vi "Cycle_Diag_Table_Read.vi"(7 "ERD Data In":T3[](array[typedef]) {"ERD Number" format="%.0x"}, 11 "error in (no error)":errorcluster) -> (2 "Cycle Buffer Status":T2, 3 "Diag Cycle String Out":string[][](array[string]), 8 "Cycle  Diag Array Out":T1[](array[typedef]), 15 "error out":errorcluster)   [LabVIEW 2021]
uses:
  Common/LabVIEW GEA2 Toolkit/GEA3/type defs/ERD Read Data Out.ctl
  type defs/Cycle_Diag_Buffer_Status.ctl
  type defs/Cycle_Diag.ctl
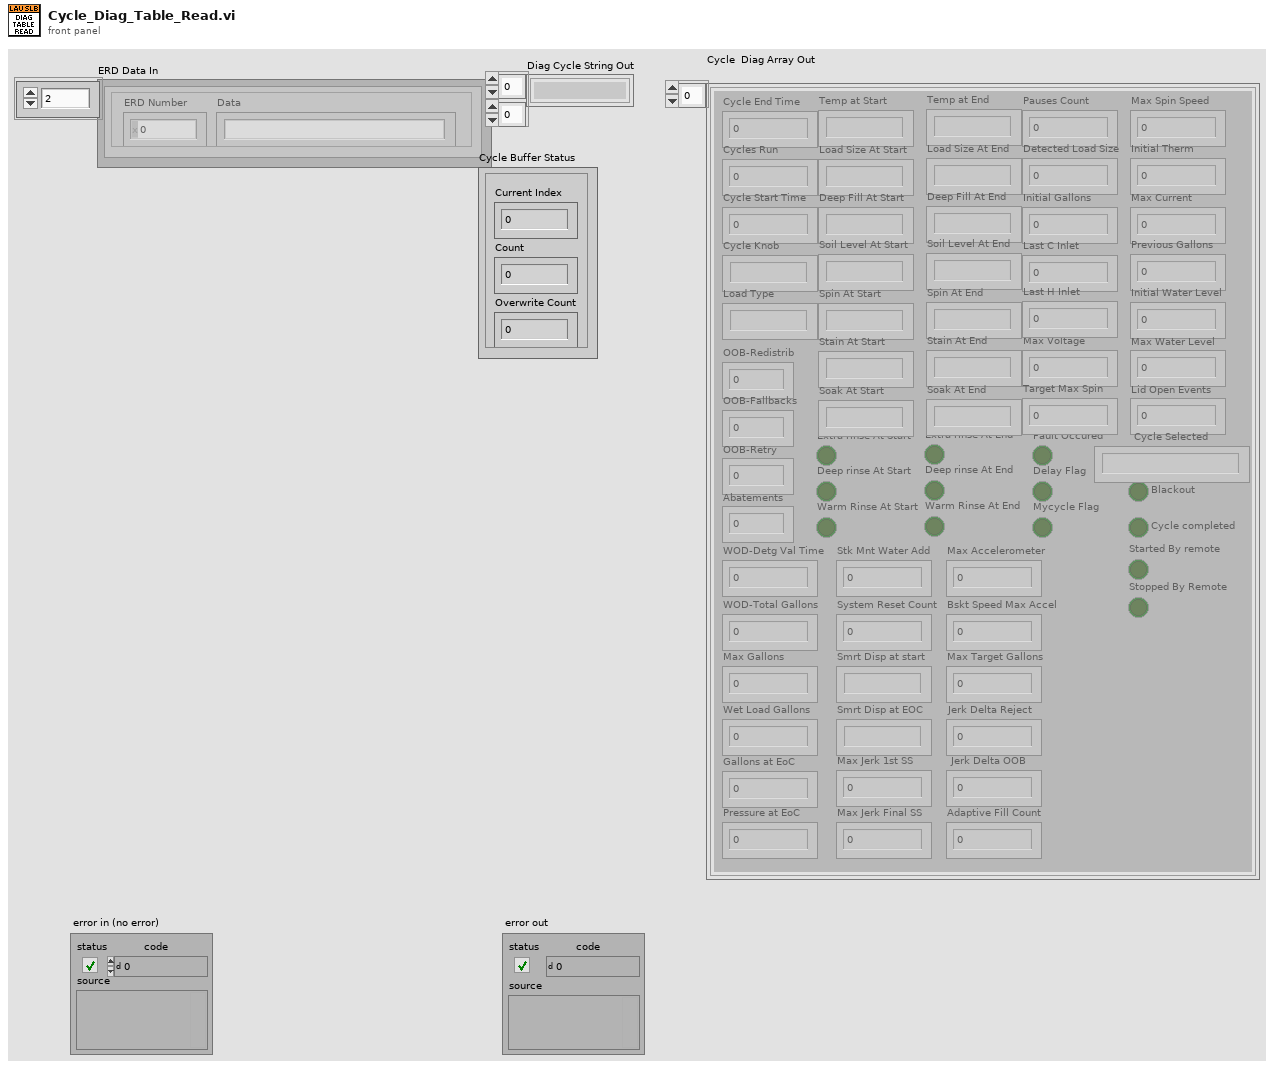
[diagram p1: front panel]
types:
  T1 = typedef "Cycle_Diag.ctl" = cluster{"Cycle End Time":u32, "Cycles Run":u32, "Cycle Start Time":u32, "Cycle Knob":string, "Load Type":string, "OOB-Redistrib":u8, "OOB-Fallbacks":u8, "OOB-Retry":u8, "Temp at Start":string, "Load Size At Start":string, "Deep Fill At Start":string, "Soil Level At Start":string, "Spin At Start":string, "Extra rinse At Start":bool, "Deep rinse At Start":bool, "Stain At Start":string, "Soak At Start":string, "Warm Rinse At Start":bool, "Temp at End":string, "Load Size At End":string, "Deep Fill At End":string, "Soil Level At End":string, "Spin At End":string, "Extra rinse At End":bool, "Deep rinse At End":bool, "Stain At End":string, "Soak At End":string, "Warm Rinse At End":bool, "Pauses Count":u8, "Fault Occured":bool, "Delay Flag":bool, "Mycycle Flag":bool, "Blackout":bool, "Cycle completed":bool, "Detected Load Size":dbl, "Initial Gallons":dbl, "Last C Inlet ":dbl, "Max Voltage":dbl, "Target Max Spin":u16, "Max Spin Speed":u16, "Initial Therm":dbl, "Max Current":dbl, "Previous Gallons":dbl, "Initial Water Level":dbl, "Max Water Level":dbl, "Abatements ":u8, "Lid Open Events":u8, "Cycle Selected":string, "Last H Inlet ":dbl, "WOD-Detg Val Time":u8, "WOD-Total Gallons":u16, "Max Gallons":u16, "Wet Load Gallons":u16, "Gallons at EoC":u16, "Pressure at EoC":u32, "Stk Mnt Water Add":u8, "Started By remote":bool, "Stopped By Remote":bool, "System Reset Count":u8, "Smrt Disp at start":string, "Smrt Disp at EOC":string, "Max Jerk 1st SS":i32, "Max Jerk Final SS":i32, "Max Accelerometer":i16, "Bskt Speed Max Accel":u16, "Max Target Gallons":u16, "Jerk Delta Reject ":u8, "Jerk Delta OOB  ":u8, "Adaptive Fill Count":u8}
  T2 = typedef "Cycle_Diag_Buffer_Status.ctl" = cluster{"Current Index":u16, "Count":u16, "Overwrite Count":u16}
  T3 = typedef "ERD Read Data Out.ctl" = cluster{"ERD Number":u16, "Data":string}
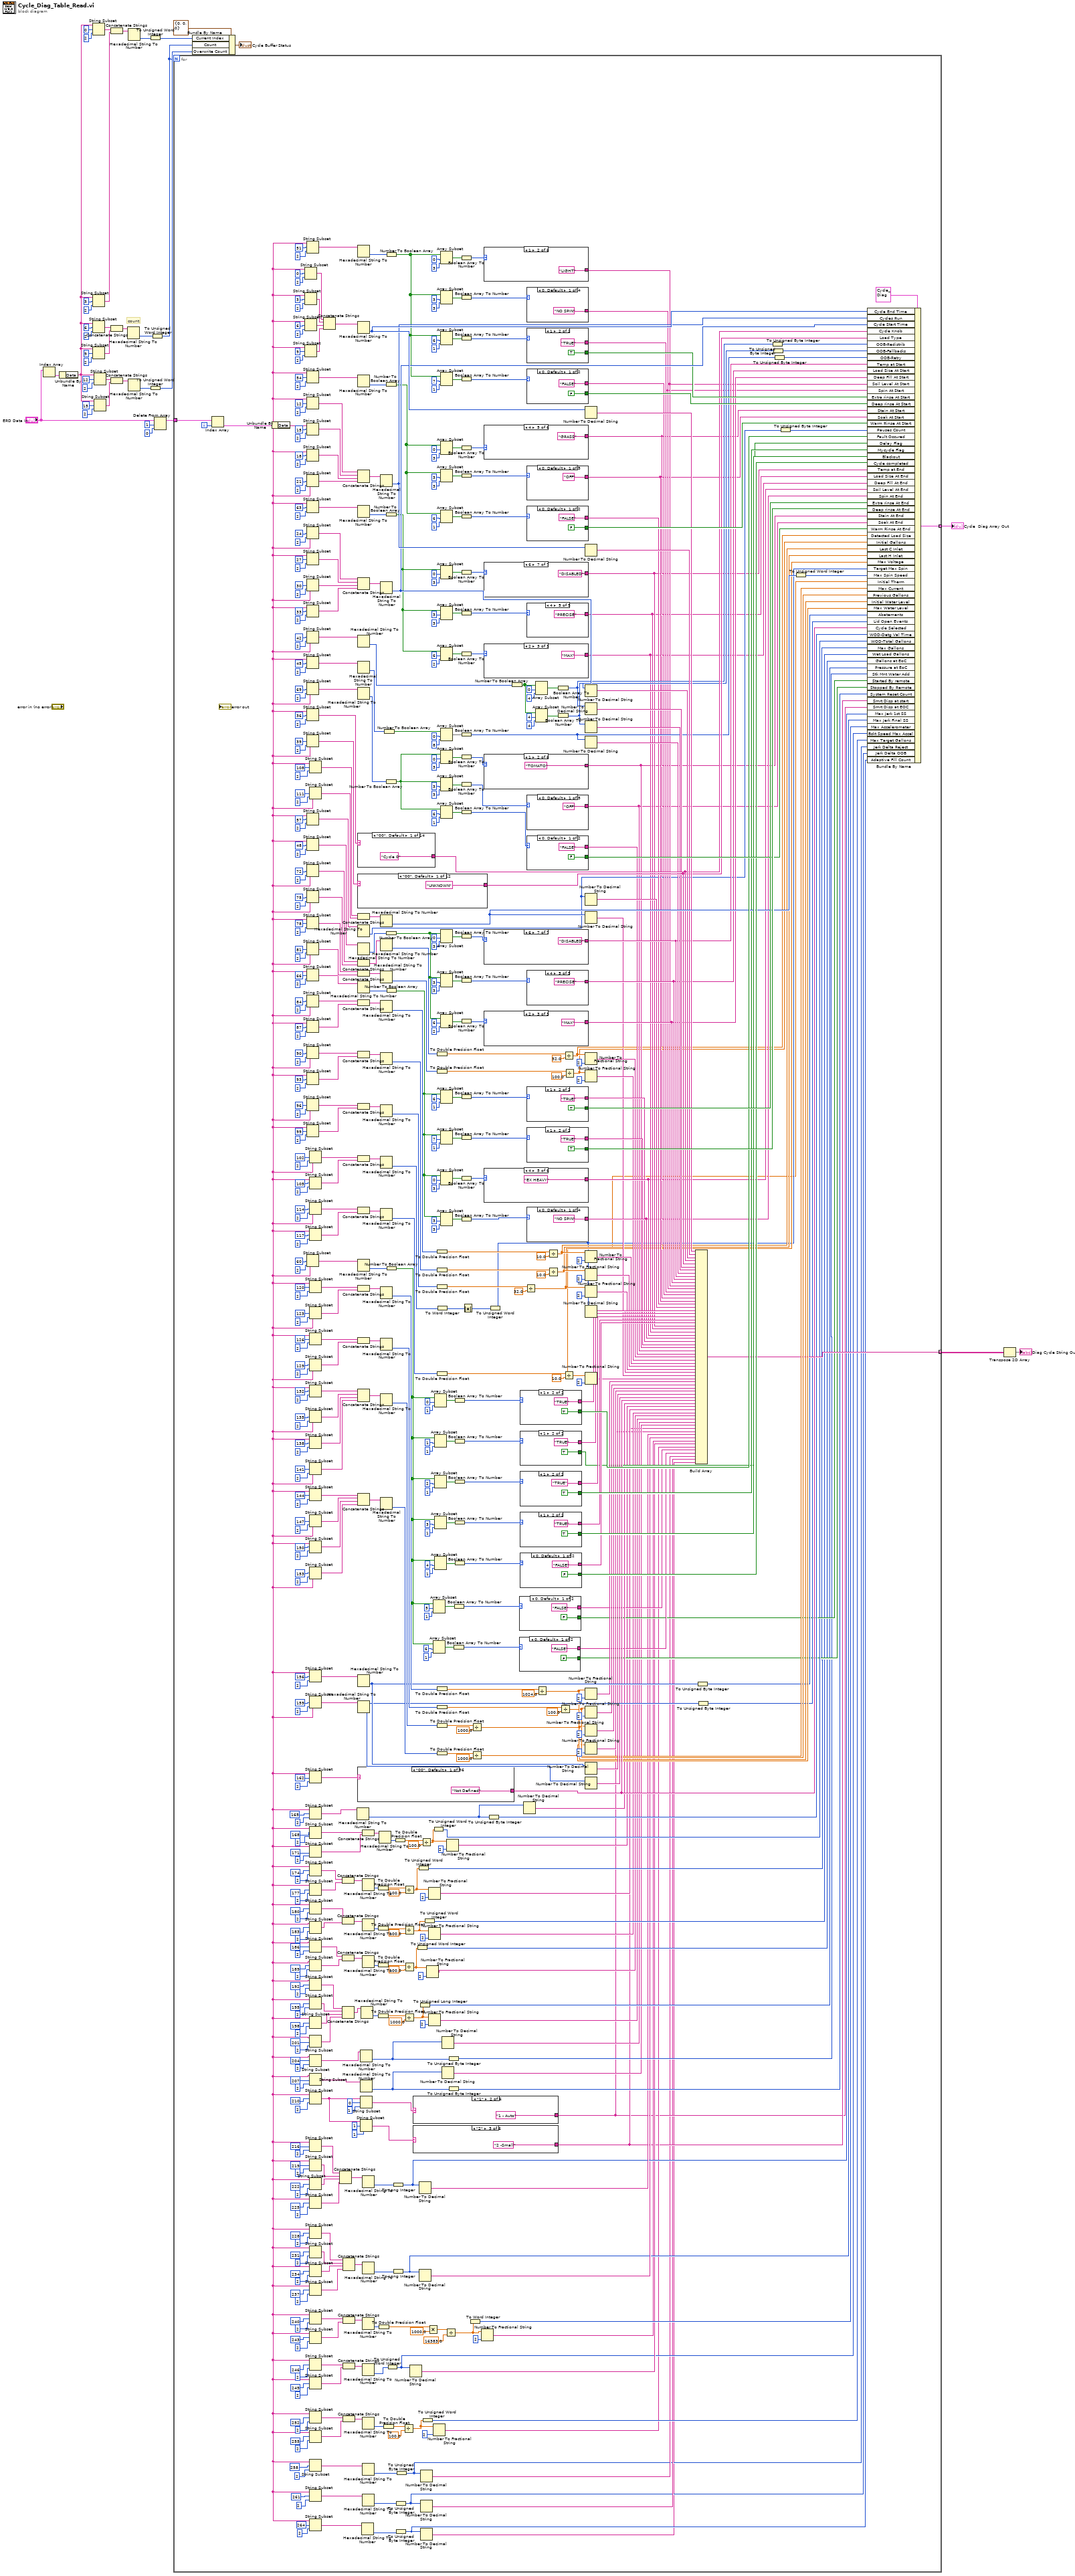
[diagram p0: block diagram]
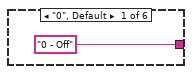
[diagram p2: hidden frame]
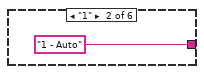
[diagram p3: hidden frame]
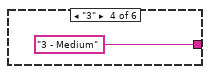
[diagram p4: hidden frame]
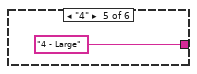
[diagram p5: hidden frame]
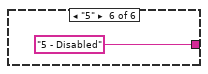
[diagram p6: hidden frame]
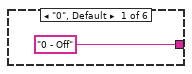
[diagram p7: hidden frame]
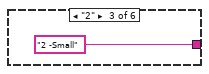
[diagram p8: hidden frame]
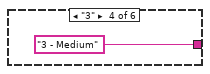
[diagram p9: hidden frame]
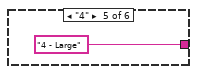
[diagram p10: hidden frame]
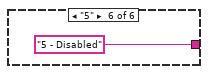
[diagram p11: hidden frame]
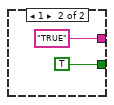
[diagram p12: hidden frame]
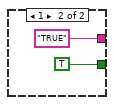
[diagram p13: hidden frame]
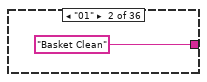
[diagram p14: hidden frame]
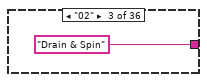
[diagram p15: hidden frame]
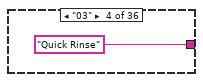
[diagram p16: hidden frame]
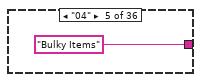
[diagram p17: hidden frame]
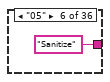
[diagram p18: hidden frame]
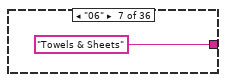
[diagram p19: hidden frame]
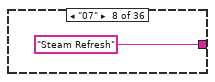
[diagram p20: hidden frame]
diagram:
  # "count"
  n1 = Index Array(array="ERD Data In") -> (element=w31:T3)  [unwired: 1 in]
  n2 = Unbundle By Name(w31) -> ("Data"=w11:string)
  n3 = String Subset(string=w11, offset (0)=0, length (rest)=2 ("length (rest)")) -> (substring=w20:string)
  n4 = String Subset(string=w11, offset (0)=3, length (rest)=2 ("length (rest)")) -> (substring=w21:string)
  n5 = String Subset(string=w11, offset (0)=6, length (rest)=2 ("length (rest)")) -> (substring=w35:string)
  n6 = String Subset(string=w11, offset (0)=9, length (rest)=2 ("length (rest)")) -> (substring=w34:string)
  n7 = String Subset(string=w11, offset (0)=12, length (rest)=2 ("length (rest)")) -> (substring=w22:string)
  n8 = String Subset(string=w11, offset (0)=15, length (rest)=2 ("length (rest)")) -> (substring=w23:string)
  n9 = Concatenate Strings(w20, w21) -> (w24:string)
  n10 = Concatenate Strings(w35, w34) -> (w33:string)
  n11 = Concatenate Strings(w22, w23) -> (w25:string)
  n12 = Hexadecimal String To Number(string=w33) -> (number=w32:u32)  [unwired: 2 in, 1 out]
  n13 = Hexadecimal String To Number(string=w24) -> (number=w26:u32)  [unwired: 2 in, 1 out]
  n14 = Hexadecimal String To Number(string=w25) -> (number=w27:u32)  [unwired: 2 in, 1 out]
  n15 = To Unsigned Word Integer(number=w26) -> (unsigned 16bit integer=w28:u16)
  n16 = To Unsigned Word Integer(number=w27) -> (unsigned 16bit integer=w29:u16)
  n17 = To Unsigned Word Integer(number=w32) -> (unsigned 16bit integer=w10:u16)
  n18 = Delete From Array(array="ERD Data In", length=1, index=0) -> (array with subset deleted=w7:T3[])  [unwired: 1 out]
  n19 = for {
    N: w10 -> [_]
    tunnel: w7 -> [w444]
    tunnel: [w441] -> w3 mode=indexing
    tunnel: [w379] -> w2 mode=indexing
    i -> [w443]
    n20 = Index Array(array=w444, index=w443) -> (element=w442:T3)
    n21 = Unbundle By Name(w442) -> ("Data"=w45:string)
    n22 = String Subset(string=w45, offset (0)=0, length (rest)=2 ("length (rest)")) -> (substring=w658:string)
    n23 = String Subset(string=w45, offset (0)=3, length (rest)=2 ("length (rest)")) -> (substring=w657:string)
    n24 = String Subset(string=w45, offset (0)=6, length (rest)=2 ("length (rest)")) -> (substring=w656:string)
    n25 = String Subset(string=w45, offset (0)=9, length (rest)=2 ("length (rest)")) -> (substring=w655:string)
    n26 = String Subset(string=w45, offset (0)=51, length (rest)=2 ("length (rest)")) -> (substring=w357:string)
    n27 = String Subset(string=w45, offset (0)=54, length (rest)=2 ("length (rest)")) -> (substring=w341:string)
    n28 = String Subset(string=w45, offset (0)=12, length (rest)=2 ("length (rest)")) -> (substring=w652:string)
    n29 = String Subset(string=w45, offset (0)=15, length (rest)=2 ("length (rest)")) -> (substring=w651:string)
    n30 = String Subset(string=w45, offset (0)=18, length (rest)=2 ("length (rest)")) -> (substring=w650:string)
    n31 = String Subset(string=w45, offset (0)=21, length (rest)=2 ("length (rest)")) -> (substring=w649:string)
    n32 = String Subset(string=w45, offset (0)=63, length (rest)=2 ("length (rest)")) -> (substring=w328:string)
    n33 = String Subset(string=w45, offset (0)=24, length (rest)=2 ("length (rest)")) -> (substring=w646:string)
    n34 = String Subset(string=w45, offset (0)=27, length (rest)=2 ("length (rest)")) -> (substring=w645:string)
    n35 = String Subset(string=w45, offset (0)=30, length (rest)=2 ("length (rest)")) -> (substring=w644:string)
    n36 = String Subset(string=w45, offset (0)=33, length (rest)=2 ("length (rest)")) -> (substring=w643:string)
    n37 = String Subset(string=w45, offset (0)=42, length (rest)=2 ("length (rest)")) -> (substring=w297:string)
    n38 = String Subset(string=w45, offset (0)=45, length (rest)=2 ("length (rest)")) -> (substring=w288:string)
    n39 = String Subset(string=w45, offset (0)=69, length (rest)=2 ("length (rest)")) -> (substring=w301:string)
    n40 = String Subset(string=w45, offset (0)=36, length (rest)=2 ("length (rest)")) -> (substring=w640:string)
    n41 = String Subset(string=w45, offset (0)=39, length (rest)=2 ("length (rest)")) -> (substring=w639:string)
    n42 = String Subset(string=w45, offset (0)=57, length (rest)=2 ("length (rest)")) -> (substring=w597:string)
    n43 = String Subset(string=w45, offset (0)=48, length (rest)=2 ("length (rest)")) -> (substring=w376:string)
    n44 = String Subset(string=w45, offset (0)=72, length (rest)=2 ("length (rest)")) -> (substring=w581:string)
    n45 = String Subset(string=w45, offset (0)=75 ("offset"), length (rest)=u32 2 ("default (0 U32)")) -> (substring=w578:string)
    n46 = String Subset(string=w45, offset (0)=78, length (rest)=2 ("length (rest)")) -> (substring=w573:string)
    n47 = String Subset(string=w45, offset (0)=81, length (rest)=2 ("length (rest)")) -> (substring=w572:string)
    n48 = String Subset(string=w45, offset (0)=66, length (rest)=2 ("length (rest)")) -> (substring=w314:string)
    n49 = String Subset(string=w45, offset (0)=84, length (rest)=2 ("length (rest)")) -> (substring=w562:string)
    n50 = String Subset(string=w45, offset (0)=87, length (rest)=2 ("length (rest)")) -> (substring=w561:string)
    n51 = String Subset(string=w45, offset (0)=90, length (rest)=2 ("length (rest)")) -> (substring=w556:string)
    n52 = String Subset(string=w45, offset (0)=93, length (rest)=2 ("length (rest)")) -> (substring=w555:string)
    n53 = String Subset(string=w45, offset (0)=96, length (rest)=2 ("length (rest)")) -> (substring=w546:string)
    n54 = String Subset(string=w45, offset (0)=99, length (rest)=2 ("length (rest)")) -> (substring=w545:string)
    n55 = String Subset(string=w45, offset (0)=60, length (rest)=2 ("length (rest)")) -> (substring=w596:string)
    n56 = String Subset(string=w45, offset (0)=108, length (rest)=2 ("length (rest)")) -> (substring=w533:string)
    n57 = String Subset(string=w45, offset (0)=111, length (rest)=2 ("length (rest)")) -> (substring=w532:string)
    n58 = String Subset(string=w45, offset (0)=102, length (rest)=2 ("length (rest)")) -> (substring=w536:string)
    n59 = String Subset(string=w45, offset (0)=105, length (rest)=2 ("length (rest)")) -> (substring=w535:string)
    n60 = String Subset(string=w45, offset (0)=114, length (rest)=2 ("length (rest)")) -> (substring=w521:string)
    n61 = String Subset(string=w45, offset (0)=117, length (rest)=2 ("length (rest)")) -> (substring=w520:string)
    n62 = String Subset(string=w45, offset (0)=120, length (rest)=2 ("length (rest)")) -> (substring=w511:string)
    n63 = String Subset(string=w45, offset (0)=123, length (rest)=2 ("length (rest)")) -> (substring=w510:string)
    n64 = String Subset(string=w45, offset (0)=126, length (rest)=2 ("length (rest)")) -> (substring=w501:string)
    n65 = String Subset(string=w45, offset (0)=129, length (rest)=2 ("length (rest)")) -> (substring=w500:string)
    n66 = String Subset(string=w45, offset (0)=132, length (rest)=2 ("length (rest)")) -> (substring=w491:string)
    n67 = String Subset(string=w45, offset (0)=135, length (rest)=2 ("length (rest)")) -> (substring=w490:string)
    n68 = String Subset(string=w45, offset (0)=138, length (rest)=2 ("length (rest)")) -> (substring=w460:string)
    n69 = String Subset(string=w45, offset (0)=141, length (rest)=2 ("length (rest)")) -> (substring=w459:string)
    n70 = String Subset(string=w45, offset (0)=144, length (rest)=2 ("length (rest)")) -> (substring=w485:string)
    n71 = String Subset(string=w45, offset (0)=147, length (rest)=2 ("length (rest)")) -> (substring=w484:string)
    n72 = String Subset(string=w45, offset (0)=150, length (rest)=2 ("length (rest)")) -> (substring=w454:string)
    n73 = String Subset(string=w45, offset (0)=153, length (rest)=2 ("length (rest)")) -> (substring=w453:string)
    n74 = String Subset(string=w45, offset (0)=156, length (rest)=2 ("length (rest)")) -> (substring=w465:string)
    n75 = String Subset(string=w45, offset (0)=159, length (rest)=2 ("length (rest)")) -> (substring=w464:string)
    n76 = String Subset(string=w45, offset (0)=162, length (rest)=2 ("length (rest)")) -> (substring=w461:string)
    n77 = String Subset(string=w45, offset (0)=165 ("length (rest)"), length (rest)=2 ("length (rest)")) -> (substring=w188:string)
    n78 = String Subset(string=w45, offset (0)=168 ("length (rest)"), length (rest)=2 ("length (rest)")) -> (substring=w172:string)
    n79 = String Subset(string=w45, offset (0)=171 ("length (rest)"), length (rest)=2 ("length (rest)")) -> (substring=w171:string)
    n80 = String Subset(string=w45, offset (0)=174 ("length (rest)"), length (rest)=2 ("length (rest)")) -> (substring=w160:string)
    n81 = String Subset(string=w45, offset (0)=177 ("length (rest)"), length (rest)=2 ("length (rest)")) -> (substring=w159:string)
    n82 = String Subset(string=w45, offset (0)=180 ("length (rest)"), length (rest)=2 ("length (rest)")) -> (substring=w149:string)
    n83 = String Subset(string=w45, offset (0)=183 ("length (rest)"), length (rest)=2 ("length (rest)")) -> (substring=w148:string)
    n84 = String Subset(string=w45, offset (0)=186 ("length (rest)"), length (rest)=2 ("length (rest)")) -> (substring=w147:string)
    n85 = String Subset(string=w45, offset (0)=189 ("length (rest)"), length (rest)=2 ("length (rest)")) -> (substring=w146:string)
    n86 = String Subset(string=w45, offset (0)=192 ("length (rest)"), length (rest)=2 ("length (rest)")) -> (substring=w144:string)
    n87 = String Subset(string=w45, offset (0)=195 ("length (rest)"), length (rest)=2 ("length (rest)")) -> (substring=w143:string)
    n88 = String Subset(string=w45, offset (0)=198 ("length (rest)"), length (rest)=2 ("length (rest)")) -> (substring=w142:string)
    n89 = String Subset(string=w45, offset (0)=201 ("length (rest)"), length (rest)=2 ("length (rest)")) -> (substring=w141:string)
    n90 = String Subset(string=w45, offset (0)=204 ("length (rest)"), length (rest)=2 ("length (rest)")) -> (substring=w134:string)
    n91 = String Subset(string=w45, offset (0)=207 ("length (rest)"), length (rest)=2 ("length (rest)")) -> (substring=w129:string)
    n92 = String Subset(string=w45, offset (0)=210 ("length (rest)"), length (rest)=2 ("length (rest)")) -> (substring=w126:string)
    n93 = String Subset(string=w45, offset (0)=216 ("length (rest)"), length (rest)=2 ("length (rest)")) -> (substring=w119:string)
    n94 = String Subset(string=w45, offset (0)=219 ("length (rest)"), length (rest)=2 ("length (rest)")) -> (substring=w118:string)
    n95 = String Subset(string=w45, offset (0)=222 ("length (rest)"), length (rest)=2 ("length (rest)")) -> (substring=w117:string)
    n96 = String Subset(string=w45, offset (0)=225 ("length (rest)"), length (rest)=2 ("length (rest)")) -> (substring=w116:string)
    n97 = String Subset(string=w45, offset (0)=228 ("length (rest)"), length (rest)=2 ("length (rest)")) -> (substring=w110:string)
    n98 = String Subset(string=w45, offset (0)=231 ("length (rest)"), length (rest)=2 ("length (rest)")) -> (substring=w109:string)
    n99 = String Subset(string=w45, offset (0)=234 ("length (rest)"), length (rest)=2 ("length (rest)")) -> (substring=w108:string)
    n100 = String Subset(string=w45, offset (0)=237 ("length (rest)"), length (rest)=2 ("length (rest)")) -> (substring=w107:string)
    n101 = String Subset(string=w45, offset (0)=240 ("length (rest)"), length (rest)=2 ("length (rest)")) -> (substring=w102:string)
    n102 = String Subset(string=w45, offset (0)=243 ("length (rest)"), length (rest)=2 ("length (rest)")) -> (substring=w101:string)
    n103 = String Subset(string=w45, offset (0)=246 ("length (rest)"), length (rest)=2 ("length (rest)")) -> (substring=w100:string)
    n104 = String Subset(string=w45, offset (0)=249 ("length (rest)"), length (rest)=2 ("length (rest)")) -> (substring=w99:string)
    n105 = String Subset(string=w45, offset (0)=252 ("length (rest)"), length (rest)=2 ("length (rest)")) -> (substring=w98:string)
    n106 = String Subset(string=w45, offset (0)=255 ("length (rest)"), length (rest)=2 ("length (rest)")) -> (substring=w97:string)
    n107 = String Subset(string=w45, offset (0)=258, length (rest)=2 ("length (rest)")) -> (substring=w50:string)
    n108 = String Subset(string=w45, offset (0)=261, length (rest)=2 ("length (rest)")) -> (substring=w53:string)
    n109 = String Subset(string=w45, offset (0)=264, length (rest)=2 ("length (rest)")) -> (substring=w42:string)
    n110 = Concatenate Strings(w658, w657, w656, w655) -> (w654:string)
    n111 = Concatenate Strings(w119, w118, w117, w116) -> (w114:string)
    n112 = Concatenate Strings(w160, w159) -> (w164:string)
    n113 = Concatenate Strings(w149, w148) -> (w157:string)
    n114 = Concatenate Strings(w147, w146) -> (w153:string)
    n115 = Concatenate Strings(w144, w143, w142, w141) -> (w137:string)
    n116 = Concatenate Strings(w110, w109, w108, w107) -> (w106:string)
    n117 = Concatenate Strings(w102, w101) -> (w95:string)
    n118 = Concatenate Strings(w100, w99) -> (w89:string)
    n119 = Concatenate Strings(w98, w97) -> (w85:string)
    n120 = Hexadecimal String To Number(string=w188) -> (number=w186:u32)  [unwired: 2 in, 1 out]
    n121 = Hexadecimal String To Number(string=w357) -> (number=w364:u32)  [unwired: 2 in, 1 out]
    n122 = Hexadecimal String To Number(string=w654) -> (number=w653:u32)  [unwired: 2 in, 1 out]
    n123 = Hexadecimal String To Number(string=w341) -> (number=w349:u32)  [unwired: 2 in, 1 out]
    n124 = Concatenate Strings(w652, w651, w650, w649) -> (w648:string)
    n125 = Hexadecimal String To Number(string=w328) -> (number=w336:u32)  [unwired: 2 in, 1 out]
    n126 = Concatenate Strings(w646, w645, w644, w643) -> (w642:string)
    n127 = Hexadecimal String To Number(string=w297) -> (number=w296:u32)  [unwired: 2 in, 1 out]
    n128 = Hexadecimal String To Number(string=w288) -> (number=w287:u32)  [unwired: 2 in, 1 out]
    n129 = Hexadecimal String To Number(string=w301) -> (number=w309:u32)  [unwired: 2 in, 1 out]
    n130 = case shown="\"00\", Default" w640 {
      tunnel: ["Cycle 0" "Cycle 1" "Cycle 2" "Cycle 3" "Cycle 4" "Cycle 5" "Cycle 6" "Cycle 7" "Cycle 8" "Cycle 9" "Cycle 10" "Cycle 11" "Cycle 12" "Cycle 13"] -> w437
      frame "00", Default {
      }
      frame "01" {
      }
      frame "02" {
      }
      frame "03" {
      }
      frame "04" {
      }
      frame "05" {
      }
      frame "06" {
      }
      frame "07" {
      }
      frame "08" {
      }
      frame "09" {
      }
      frame "0A" {
      }
      frame "0B" {
      }
      frame "0C" {
      }
      frame "0D" {
      }
    }
    n131 = case shown="\"00\", Default" w639 {
      tunnel: ["UNKNOWN" "COTTON" "SYNTHETIC" "MIXED" "WET" "LOW FLOW" "SMALL" "MEDIUM" "LARGE" "SUPER" "SUPER PLUS" "MAX"] -> w436
      frame "00", Default {
      }
      frame "01" {
      }
      frame "02" {
      }
      frame "03" {
      }
      frame "04" {
      }
      frame "05" {
      }
      frame "06" {
      }
      frame "07" {
      }
      frame "08" {
      }
      frame "09" {
      }
      frame "0A" {
      }
      frame "0B" {
      }
    }
    n132 = Concatenate Strings(w533, w532) -> (w531:string)
    n133 = Hexadecimal String To Number(string=w597) -> (number=w420:u32)  [unwired: 2 in, 1 out]
    n134 = Hexadecimal String To Number(string=w376) -> (number=w375:u32)  [unwired: 2 in, 1 out]
    n135 = Concatenate Strings(w581, w578) -> (w577:string)
    n136 = Concatenate Strings(w573, w572) -> (w571:string)
    n137 = Hexadecimal String To Number(string=w314) -> (number=w324:u32)  [unwired: 2 in, 1 out]
    n138 = Concatenate Strings(w562, w561) -> (w560:string)
    n139 = Concatenate Strings(w556, w555) -> (w554:string)
    n140 = Concatenate Strings(w546, w545) -> (w544:string)
    n141 = Concatenate Strings(w536, w535) -> (w534:string)
    n142 = Concatenate Strings(w521, w520) -> (w519:string)
    n143 = Hexadecimal String To Number(string=w596) -> (number=w595:u32)  [unwired: 2 in, 1 out]
    n144 = Concatenate Strings(w511, w510) -> (w509:string)
    n145 = Concatenate Strings(w501, w500) -> (w499:string)
    n146 = Concatenate Strings(w491, w490, w460, w459) -> (w489:string)
    n147 = Concatenate Strings(w485, w484, w454, w453) -> (w483:string)
    n148 = Hexadecimal String To Number(string=w465) -> (number=w463:u32)  [unwired: 2 in, 1 out]
    n149 = Hexadecimal String To Number(string=w464) -> (number=w462:u32)  [unwired: 2 in, 1 out]
    n150 = case shown="\"00\", Default" w461 {
      tunnel: ["Not Defined" "Basket Clean" "Drain & Spin" "Quick Rinse" "Bulky Items" "Sanitize" "Towels & Sheets" "Steam Refresh" "Normal/Mixed" "Whites" "Dark Colors" "Jeans" "Hand Wash" "Delicates" "Speed Wash" "Heavy Duty" "Allergen" "Power Clean" "Rinse & Spin" "Single Item" "Colors" "Cold Wash" "Cottons" "Easy Care" "Active Wear" "Timed Dry" "Dewrinkle" "Air Fluff" "Steam Refresh" "Steam Dewrinkle" "Speed Dry" "Mixed" "Quick Dry" "Casuals" "Warm Up" "Energy Saver"] -> w387
      frame "00", Default {
      }
      frame "01" {
      }
      frame "02" {
      }
      frame "03" {
      }
      frame "04" {
      }
      frame "05" {
      }
      frame "06" {
      }
      frame "07" {
      }
      frame "08" {
      }
      frame "09" {
      }
      frame "0A" {
      }
      frame "0B" {
      }
      frame "0C" {
      }
      frame "0D" {
      }
      frame "0E" {
      }
      frame "0F" {
      }
      frame "10" {
      }
      frame "11" {
      }
      frame "12" {
      }
      frame "13" {
      }
      frame "14" {
      }
      frame "15" {
      }
      frame "80" {
      }
      frame "81" {
      }
      frame "82" {
      }
      frame "83" {
      }
      frame "84" {
      }
      frame "85" {
      }
      frame "86" {
      }
      frame "87" {
      }
      frame "88" {
      }
      frame "89" {
      }
      frame "8A" {
      }
      frame "8B" {
      }
      frame "8C" {
      }
      frame "8D" {
      }
    }
    n151 = Hexadecimal String To Number(string=w134) -> (number=w133:u32)  [unwired: 2 in, 1 out]
    n152 = Hexadecimal String To Number(string=w129) -> (number=w130:u32)  [unwired: 2 in, 1 out]
    n153 = String Subset(string=w126, offset (0)=0, length (rest)=1 ("length (rest)")) -> (substring=w121:string)
    n154 = String Subset(string=w126, offset (0)=1, length (rest)=1 ("length (rest)")) -> (substring=w120:string)
    n155 = Hexadecimal String To Number(string=w137) -> (number=w140:u32)  [unwired: 2 in, 1 out]
    n156 = Hexadecimal String To Number(string=w42) -> (number=w41:u32)  [unwired: 2 in, 1 out]
    n157 = Concatenate Strings(w172, w171) -> (w170:string)
    n158 = Hexadecimal String To Number(string=w164) -> (number=w163:u32)  [unwired: 2 in, 1 out]
    n159 = Hexadecimal String To Number(string=w157) -> (number=w156:u32)  [unwired: 2 in, 1 out]
    n160 = Hexadecimal String To Number(string=w153) -> (number=w152:u32)  [unwired: 2 in, 1 out]
    n161 = Hexadecimal String To Number(string=w95) -> (number=w96:u32)  [unwired: 2 in, 1 out]
    n162 = Hexadecimal String To Number(string=w89) -> (number=w60:u32)  [unwired: 2 in, 1 out]
    n163 = Hexadecimal String To Number(string=w85) -> (number=w86:u32)  [unwired: 2 in, 1 out]
    n164 = Hexadecimal String To Number(string=w50) -> (number=w52:u32)  [unwired: 2 in, 1 out]
    n165 = Hexadecimal String To Number(string=w53) -> (number=w51:u32)  [unwired: 2 in, 1 out]
    n166 = Hexadecimal String To Number(string=w114) -> (number=w113:u32)  [unwired: 2 in, 1 out]
    n167 = Hexadecimal String To Number(string=w106) -> (number=w105:u32)  [unwired: 2 in, 1 out]
    n168 = To Double Precision Float(number=w163) -> (double precision float=w162:dbl)
    n169 = To Double Precision Float(number=w156) -> (double precision float=w155:dbl)
    n170 = To Double Precision Float(number=w152) -> (double precision float=w151:dbl)
    n171 = To Double Precision Float(number=w140) -> (double precision float=w139:dbl)
    n172 = To Double Precision Float(number=w96) -> (double precision float=w94:dbl)
    n173 = Hexadecimal String To Number(string=w170) -> (number=w169:u32)  [unwired: 2 in, 1 out]
    n174 = Hexadecimal String To Number(string=w648) -> (number=w647:u32)  [unwired: 2 in, 1 out]
    n175 = Hexadecimal String To Number(string=w642) -> (number=w641:u32)  [unwired: 2 in, 1 out]
    n176 = Hexadecimal String To Number(string=w531) -> (number=w530:u32)  [unwired: 2 in, 1 out]
    n177 = Hexadecimal String To Number(string=w577) -> (number=w584:u32)  [unwired: 2 in, 1 out]
    n178 = Hexadecimal String To Number(string=w571) -> (number=w570:u32)  [unwired: 2 in, 1 out]
    n179 = Hexadecimal String To Number(string=w560) -> (number=w559:u32)  [unwired: 2 in, 1 out]
    n180 = Hexadecimal String To Number(string=w554) -> (number=w553:u32)  [unwired: 2 in, 1 out]
    n181 = Hexadecimal String To Number(string=w544) -> (number=w543:u32)  [unwired: 2 in, 1 out]
    n182 = Hexadecimal String To Number(string=w534) -> (number=w446:u32)  [unwired: 2 in, 1 out]
    n183 = Hexadecimal String To Number(string=w519) -> (number=w518:u32)  [unwired: 2 in, 1 out]
    n184 = Hexadecimal String To Number(string=w509) -> (number=w508:u32)  [unwired: 2 in, 1 out]
    n185 = Hexadecimal String To Number(string=w499) -> (number=w498:u32)  [unwired: 2 in, 1 out]
    n186 = Hexadecimal String To Number(string=w489) -> (number=w488:u32)  [unwired: 2 in, 1 out]
    n187 = Hexadecimal String To Number(string=w483) -> (number=w482:u32)  [unwired: 2 in, 1 out]
    n188 = To Double Precision Float(number=w86) -> (double precision float=w84:dbl)
    n189 = Number To Boolean Array(number=w287) -> (Boolean array=w286:bool[])
    n190 = Number To Boolean Array(number=w349) -> (Boolean array=w348:bool[])
    n191 = Number To Boolean Array(number=w336) -> (Boolean array=w335:bool[])
    n192 = Number To Boolean Array(number=w309) -> (Boolean array=w308:bool[])
    n193 = Number To Boolean Array(number=w375) -> (Boolean array=w374:bool[])
    n194 = Number To Boolean Array(number=w364) -> (Boolean array=w356:bool[])
    n195 = Number To Boolean Array(number=w324) -> (Boolean array=w317:bool[])
    n196 = Number To Boolean Array(number=w595) -> (Boolean array=w176:bool[])
    n197 = To Unsigned Word Integer(number=w60) -> (unsigned 16bit integer=w87:u16)
    n198 = To Long Integer(number=w113) -> (32bit integer=w111:i32)
    n199 = To Long Integer(number=w105) -> (32bit integer=w103:i32)
    n200 = To Double Precision Float(number=w169) -> (double precision float=w168:dbl)
    n201 = To Unsigned Byte Integer(number=w51) -> (unsigned 8bit integer=w46:u8)
    n202 = To Unsigned Byte Integer(number=w41) -> (unsigned 8bit integer=w40:u8)
    n203 = To Unsigned Byte Integer(number=w52) -> (unsigned 8bit integer=w47:u8)
    n204 = Divide(x=w84, y=100.0) -> (x/y=w68:dbl)
    n205 = Divide(x=w162, y=100.0) -> (x/y=w79:dbl)
    n206 = Divide(x=w155, y=100.0) -> (x/y=w76:dbl)
    n207 = Divide(x=w151, y=100.0) -> (x/y=w75:dbl)
    n208 = Divide(x=w139, y=1000.0) -> (x/y=w72:dbl)
    n209 = Number To Decimal String(number=w87) -> (decimal integer string=w88:string)  [unwired: 1 in]
    n210 = case shown="\"2\"" w120 {
      tunnel: ["0 - Off" "1 - Auto" "2 -Small" "3 - Medium" "4 - Large" "5 - Disabled"] -> w59
      frame "0", Default {
      }
      frame "1" {
      }
      frame "2" {
      }
      frame "3" {
      }
      frame "4" {
      }
      frame "5" {
      }
    }
    n211 = case shown="\"1\"" w121 {
      tunnel: ["0 - Off" "1 - Auto" "2 -Small" "3 - Medium" "4 - Large" "5 - Disabled"] -> w58
      frame "0", Default {
      }
      frame "1" {
      }
      frame "2" {
      }
      frame "3" {
      }
      frame "4" {
      }
      frame "5" {
      }
    }
    n212 = To Unsigned Word Integer(number=w75) -> (unsigned 16bit integer=w135:u16)
    n213 = To Unsigned Word Integer(number=w79) -> (unsigned 16bit integer=w158:u16)
    n214 = To Unsigned Long Integer(number=w72) -> (unsigned 32bit integer=w136:u32)
    n215 = Number To Decimal String(number=w111) -> (decimal integer string=w112:string)  [unwired: 1 in]
    n216 = Number To Decimal String(number=w103) -> (decimal integer string=w104:string)  [unwired: 1 in]
    n217 = Number To Decimal String(number=w47) -> (decimal integer string=w49:string)  [unwired: 1 in]
    n218 = Number To Decimal String(number=w46) -> (decimal integer string=w48:string)  [unwired: 1 in]
    n219 = Number To Decimal String(number=w40) -> (decimal integer string=w39:string)  [unwired: 1 in]
    n220 = Divide(x=w168, y=100.0) -> (x/y=w81:dbl)
    n221 = To Unsigned Word Integer(number=w68) -> (unsigned 16bit integer=w82:u16)
    n222 = To Unsigned Word Integer(number=w76) -> (unsigned 16bit integer=w145:u16)
    n223 = Number To Fractional String(number=w75, precision (6)=i16 2) -> (F-format string=w74:string)  [unwired: 2 in]
    n224 = Multiply(x=w94, y=1000.0) -> (x*y=w92:dbl)
    n225 = Number To Fractional String(number=w72, precision (6)=i16 2) -> (F-format string=w73:string)  [unwired: 2 in]
    n226 = Number To Fractional String(number=w79, precision (6)=i16 2) -> (F-format string=w78:string)  [unwired: 2 in]
    n227 = Number To Fractional String(number=w76, precision (6)=i16 2) -> (F-format string=w77:string)  [unwired: 2 in]
    n228 = To Unsigned Word Integer(number=w81) -> (unsigned 16bit integer=w166:u16)
    n229 = Array Subset(array=w176, index=6, length=1) -> (w177:bool[])
    n230 = Number To Fractional String(number=w68, precision (6)=i16 2) -> (F-format string=w69:string)  [unwired: 2 in]
    n231 = Array Subset(array=w176, index=5, length=1) -> (w181:bool[])
    n232 = Array Subset(array=w176, index=0, length=1) -> (w272:bool[])
    n233 = Array Subset(array=w176, index=1, length=1) -> (w270:bool[])
    n234 = Array Subset(array=w176, index=2, length=1) -> (w269:bool[])
    n235 = Array Subset(array=w176, index=3, length=1) -> (w268:bool[])
    n236 = Array Subset(array=w176, index=4, length=1) -> (w267:bool[])
    n237 = To Double Precision Float(number=w584) -> (double precision float=w583:dbl)
    n238 = To Double Precision Float(number=w570) -> (double precision float=w569:dbl)
    n239 = To Double Precision Float(number=w559) -> (double precision float=w558:dbl)
    n240 = To Double Precision Float(number=w553) -> (double precision float=w552:dbl)
    n241 = To Double Precision Float(number=w543) -> (double precision float=w542:dbl)
    n242 = To Word Integer(number=w446) -> (16bit integer=w448:i16)
    n243 = To Double Precision Float(number=w518) -> (double precision float=w517:dbl)
    n244 = To Double Precision Float(number=w508) -> (double precision float=w507:dbl)
    n245 = To Double Precision Float(number=w498) -> (double precision float=w497:dbl)
    n246 = To Double Precision Float(number=w488) -> (double precision float=w487:dbl)
    n247 = To Double Precision Float(number=w482) -> (double precision float=w481:dbl)
    n248 = Array Subset(array=w356, index=0, length=3) -> (w353:bool[])
    n249 = Array Subset(array=w356, index=3, length=3) -> (w352:bool[])
    n250 = Array Subset(array=w356, index=6, length=1) -> (w351:bool[])
    n251 = Array Subset(array=w356, index=7, length=1) -> (w350:bool[])
    n252 = Array Subset(array=w348, index=0, length=3) -> (w339:bool[])
    n253 = Array Subset(array=w348, index=3, length=3) -> (w338:bool[])
    n254 = Array Subset(array=w348, index=6, length=1) -> (w337:bool[])
    n255 = Array Subset(array=w335, index=0, length=3) -> (w327:bool[])
    n256 = Array Subset(array=w335, index=3, length=3) -> (w326:bool[])
    n257 = Array Subset(array=w335, index=6, length=2) -> (w325:bool[])
    n258 = Array Subset(array=w286, index=0, length=8) -> (w283:bool[])
    n259 = Array Subset(array=w308, index=0, length=3) -> (w300:bool[])
    n260 = Array Subset(array=w308, index=3, length=3) -> (w299:bool[])
    n261 = Array Subset(array=w308, index=6, length=1) -> (w298:bool[])
    n262 = Array Subset(array=w374, index=0, length=3) -> (w367:bool[])
    n263 = Array Subset(array=w374, index=3, length=3) -> (w366:bool[])
    n264 = Array Subset(array=w374, index=6, length=2) -> (w365:bool[])
    n265 = Array Subset(array=w317, index=6, length=1) -> (w311:bool[])
    n266 = Array Subset(array=w317, index=7, length=1) -> (w310:bool[])
    n267 = Array Subset(array=w317, index=0, length=3) -> (w313:bool[])
    n268 = Array Subset(array=w317, index=3, length=3) -> (w312:bool[])
    n269 = Number To Decimal String(number=w133) -> (decimal integer string=w132:string)  [unwired: 1 in]
    n270 = Number To Decimal String(number=w130) -> (decimal integer string=w128:string)  [unwired: 1 in]
    n271 = Divide(x=w92, y=16383.0) -> (x/y=w70:dbl)
    n272 = Number To Fractional String(number=w81, precision (6)=i16 2) -> (F-format string=w80:string)  [unwired: 2 in]
    n273 = To Unsigned Byte Integer(number=w133) -> (unsigned 8bit integer=w131:u8)
    n274 = To Unsigned Byte Integer(number=w130) -> (unsigned 8bit integer=w127:u8)
    n275 = Boolean Array To Number(Boolean array=w177) -> (number=w180:u32)
    n276 = Boolean Array To Number(Boolean array=w181) -> (number=w184:u32)
    n277 = Boolean Array To Number(Boolean array=w272) -> (number=w594:u32)
    n278 = Boolean Array To Number(Boolean array=w270) -> (number=w593:u32)
    n279 = Boolean Array To Number(Boolean array=w269) -> (number=w592:u32)
    n280 = Boolean Array To Number(Boolean array=w268) -> (number=w591:u32)
    n281 = Boolean Array To Number(Boolean array=w267) -> (number=w590:u32)
    n282 = Boolean Array To Number(Boolean array=w353) -> (number=w630:u32)
    n283 = Boolean Array To Number(Boolean array=w352) -> (number=w629:u32)
    n284 = Boolean Array To Number(Boolean array=w351) -> (number=w628:u32)
    n285 = Boolean Array To Number(Boolean array=w350) -> (number=w627:u32)
    n286 = Boolean Array To Number(Boolean array=w339) -> (number=w624:u32)
    n287 = Boolean Array To Number(Boolean array=w338) -> (number=w623:u32)
    n288 = Boolean Array To Number(Boolean array=w337) -> (number=w622:u32)
    n289 = Boolean Array To Number(Boolean array=w327) -> (number=w614:u32)
    n290 = Boolean Array To Number(Boolean array=w326) -> (number=w613:u32)
    n291 = Boolean Array To Number(Boolean array=w325) -> (number=w612:u32)
    n292 = Boolean Array To Number(Boolean array=w283) -> (number=w430:u32)
    n293 = Boolean Array To Number(Boolean array=w300) -> (number=w607:u32)
    n294 = Boolean Array To Number(Boolean array=w299) -> (number=w606:u32)
    n295 = Boolean Array To Number(Boolean array=w298) -> (number=w605:u32)
    n296 = Boolean Array To Number(Boolean array=w367) -> (number=w445:u32)
    n297 = Boolean Array To Number(Boolean array=w366) -> (number=w632:u32)
    n298 = Boolean Array To Number(Boolean array=w365) -> (number=w631:u32)
    n299 = Boolean Array To Number(Boolean array=w311) -> (number=w609:u32)
    n300 = Boolean Array To Number(Boolean array=w310) -> (number=w608:u32)
    n301 = Boolean Array To Number(Boolean array=w313) -> (number=w611:u32)
    n302 = Boolean Array To Number(Boolean array=w312) -> (number=w610:u32)
    n303 = Absolute Value(x=w448) -> (abs(x)=w447:i16)
    n304 = To Word Integer(number=w70) -> (16bit integer=w90:i16)
    n305 = Divide(x=w487, y=1000.0) -> (x/y=w381:dbl)
    n306 = Divide(x=w481, y=1000.0) -> (x/y=w380:dbl)
    n307 = Number To Fractional String(number=w70, precision (6)=i16 2) -> (F-format string=w71:string)  [unwired: 2 in]
    n308 = case shown="1" w630 {
      tunnel: ["EXTRA LIGHT" "LIGHT" "NORMAL" "HEAVY" "EX HEAVY" "DISABLED"] -> w426
      frame 0, Default {
      }
      frame 1 {
      }
      frame 2 {
      }
      frame 3 {
      }
      frame 4 {
      }
      frame 5 {
      }
    }
    n309 = case shown="4" w624 {
      tunnel: ["OFF" "TOMATO" "WINE" "BLOOD" "GRASS" "DIRT"] -> w340
      frame 0, Default {
      }
      frame 1 {
      }
      frame 2 {
      }
      frame 3 {
      }
      frame 4 {
      }
      frame 5 {
      }
    }
    n310 = case shown="6" w614 {
      tunnel: ["TAP COLD" "COLD" "COOL" "COLORS" "WARM" "HOT" "DISABLED"] -> w412
      frame 0, Default {
      }
      frame 1 {
      }
      frame 2 {
      }
      frame 3 {
      }
      frame 4 {
      }
      frame 5 {
      }
      frame 6 {
      }
    }
    n311 = case shown="2" w612 {
      tunnel: ["OFF" "INCREMENTAL" "MAX"] -> w410
      frame 0, Default {
      }
      frame 1 {
      }
      frame 2 {
      }
    }
    n312 = case shown="1" w607 {
      tunnel: ["OFF" "TOMATO" "WINE" "BLOOD" "GRASS" "DIRT"] -> w405
      frame 0, Default {
      }
      frame 1 {
      }
      frame 2 {
      }
      frame 3 {
      }
      frame 4 {
      }
      frame 5 {
      }
    }
    n313 = case shown="6" w445 {
      tunnel: ["TAP COLD" "COLD" "COOL" "COLORS" "WARM" "HOT" "DISABLED"] -> w429
      frame 0, Default {
      }
      frame 1 {
      }
      frame 2 {
      }
      frame 3 {
      }
      frame 4 {
      }
      frame 5 {
      }
      frame 6 {
      }
    }
    n314 = case shown="2" w631 {
      tunnel: ["OFF" "INCREMENTAL" "MAX"] -> w427
      frame 0, Default {
      }
      frame 1 {
      }
      frame 2 {
      }
    }
    n315 = case shown="4" w611 {
      tunnel: ["EXTRA LIGHT" "LIGHT" "NORMAL" "HEAVY" "EX HEAVY" "DISABLED"] -> w409
      frame 0, Default {
      }
      frame 1 {
      }
      frame 2 {
      }
      frame 3 {
      }
      frame 4 {
      }
      frame 5 {
      }
    }
    n316 = To Unsigned Byte Integer(number=w186) -> (unsigned 8bit integer=w185:u8)
    n317 = To Unsigned Word Integer(number=w447) -> (unsigned 16bit integer=w256:u16)
    n318 = Number To Boolean Array(number=w296) -> (Boolean array=w291:bool[])
    n319 = case shown="0, Default" w180 {
      tunnel: [FALSE TRUE] -> w165
      tunnel: ["FALSE" "TRUE"] -> w174
      frame 0, Default {
      }
      frame 1 {
      }
    }
    n320 = case shown="0, Default" w184 {
      tunnel: [FALSE TRUE] -> w173
      tunnel: ["FALSE" "TRUE"] -> w175
      frame 0, Default {
      }
      frame 1 {
      }
    }
    n321 = case shown="1" w594 {
      tunnel: [FALSE TRUE] -> w589
      tunnel: ["FALSE" "TRUE"] -> w417
      frame 0, Default {
      }
      frame 1 {
      }
    }
    n322 = case shown="1" w593 {
      tunnel: [FALSE TRUE] -> w271
      tunnel: ["FALSE" "TRUE"] -> w416
      frame 0, Default {
      }
      frame 1 {
      }
    }
    n323 = case shown="1" w592 {
      tunnel: [FALSE TRUE] -> w418
      tunnel: ["FALSE" "TRUE"] -> w415
      frame 0, Default {
      }
      frame 1 {
      }
    }
    n324 = case shown="1" w591 {
      tunnel: [FALSE TRUE] -> w588
      tunnel: ["FALSE" "TRUE"] -> w414
      frame 0, Default {
      }
      frame 1 {
      }
    }
    n325 = case shown="0, Default" w590 {
      tunnel: [FALSE TRUE] -> w587
      tunnel: ["FALSE" "TRUE"] -> w413
      frame 0, Default {
      }
      frame 1 {
      }
    }
    n326 = Number To Decimal String(number=w186) -> (decimal integer string=w187:string)  [unwired: 1 in]
    n327 = Divide(x=w542, y=32.0) -> (x/y=w384:dbl)
    n328 = case shown="0, Default" w629 {
      tunnel: ["NO SPIN" "NORMAL" "MORE" "MAX"] -> w425
      frame 0, Default {
      }
      frame 1 {
      }
      frame 2 {
      }
      frame 3 {
      }
    }
    n329 = case shown="1" w628 {
      tunnel: [FALSE TRUE] -> w626
      tunnel: ["FALSE" "TRUE"] -> w424
      frame 0, Default {
      }
      frame 1 {
      }
    }
    n330 = case shown="0, Default" w627 {
      tunnel: [FALSE TRUE] -> w625
      tunnel: ["FALSE" "TRUE"] -> w423
      frame 0, Default {
      }
      frame 1 {
      }
    }
    n331 = case shown="0, Default" w623 {
      tunnel: ["OFF" "15 MIN" "30 MIN" "60 MIN" "2 HOURS"] -> w422
      frame 0, Default {
      }
      frame 1 {
      }
      frame 2 {
      }
      frame 3 {
      }
      frame 4 {
      }
    }
    n332 = case shown="0, Default" w622 {
      tunnel: [FALSE TRUE] -> w621
      tunnel: ["FALSE" "TRUE"] -> w421
      frame 0, Default {
      }
      frame 1 {
      }
    }
    n333 = case shown="4" w613 {
      tunnel: ["SMALL" "MEDIUM" "LARGE" "SUPER" "PRECISE"] -> w411
      frame 0, Default {
      }
      frame 1 {
      }
      frame 2 {
      }
      frame 3 {
      }
      frame 4 {
      }
    }
    n334 = case shown="0, Default" w606 {
      tunnel: ["OFF" "15 MIN" "30 MIN" "60 MIN" "2 HOURS"] -> w404
      frame 0, Default {
      }
      frame 1 {
      }
      frame 2 {
      }
      frame 3 {
      }
      frame 4 {
      }
    }
    n335 = case shown="0, Default" w605 {
      tunnel: [FALSE TRUE] -> w602
      tunnel: ["FALSE" "TRUE"] -> w403
      frame 0, Default {
      }
      frame 1 {
      }
    }
    n336 = case shown="4" w632 {
      tunnel: ["SMALL" "MEDIUM" "LARGE" "SUPER" "PRECISE"] -> w428
      frame 0, Default {
      }
      frame 1 {
      }
      frame 2 {
      }
      frame 3 {
      }
      frame 4 {
      }
    }
    n337 = case shown="1" w609 {
      tunnel: [FALSE TRUE] -> w604
      tunnel: ["FALSE" "TRUE"] -> w407
      frame 0, Default {
      }
      frame 1 {
      }
    }
    n338 = case shown="1" w608 {
      tunnel: [FALSE TRUE] -> w603
      tunnel: ["FALSE" "TRUE"] -> w406
      frame 0, Default {
      }
      frame 1 {
      }
    }
    n339 = case shown="0, Default" w610 {
      tunnel: ["NO SPIN" "NORMAL" "MORE" "MAX"] -> w408
      frame 0, Default {
      }
      frame 1 {
      }
      frame 2 {
      }
      frame 3 {
      }
    }
    n340 = Array Subset(array=w291, index=0, length=4) -> (w290:bool[])
    n341 = Array Subset(array=w291, index=4, length=4) -> (w289:bool[])
    n342 = Divide(x=w507, y=1024.0) -> (x/y=w383:dbl)
    n343 = Divide(x=w558, y=10.0) -> (x/y=w386:dbl)
    n344 = Divide(x=w552, y=10.0) -> (x/y=w385:dbl)
    n345 = Boolean Array To Number(Boolean array=w290) -> (number=w435:u32)
    n346 = Boolean Array To Number(Boolean array=w289) -> (number=w433:u32)
    n347 = Divide(x=w497, y=100.0) -> (x/y=w382:dbl)
    n348 = Divide(x=w583, y=32.0) -> (x/y=w402:dbl)
    n349 = Divide(x=w517, y=10.0) -> (x/y=w115:dbl)
    n350 = Divide(x=w569, y=100.0) -> (x/y=w378:dbl)
    n351 = Number To Decimal String(number=w653) -> (decimal integer string=w440:string)  [unwired: 1 in]
    n352 = Number To Decimal String(number=w647) -> (decimal integer string=w439:string)  [unwired: 1 in]
    n353 = Number To Decimal String(number=w641) -> (decimal integer string=w438:string)  [unwired: 1 in]
    n354 = Number To Decimal String(number=w435) -> (decimal integer string=w434:string)  [unwired: 1 in]
    n355 = Number To Decimal String(number=w433) -> (decimal integer string=w432:string)  [unwired: 1 in]
    n356 = Number To Decimal String(number=w430) -> (decimal integer string=w431:string)  [unwired: 1 in]
    n357 = Number To Decimal String(number=w420) -> (decimal integer string=w419:string)  [unwired: 1 in]
    n358 = Number To Decimal String(number=w530) -> (decimal integer string=w395:string)  [unwired: 1 in]
    n359 = Number To Fractional String(number=w402, precision (6)=i16 2) -> (F-format string=w401:string)  [unwired: 2 in]
    n360 = Number To Fractional String(number=w378, precision (6)=i16 2) -> (F-format string=w400:string)  [unwired: 2 in]
    n361 = Number To Fractional String(number=w386, precision (6)=i16 2) -> (F-format string=w399:string)  [unwired: 2 in]
    n362 = Number To Fractional String(number=w385, precision (6)=i16 2) -> (F-format string=w398:string)  [unwired: 2 in]
    n363 = Number To Fractional String(number=w384, precision (6)=i16 2) -> (F-format string=w397:string)  [unwired: 2 in]
    n364 = Number To Decimal String(number=w256) -> (decimal integer string=w396:string)  [unwired: 1 in]
    n365 = Number To Fractional String(number=w115, precision (6)=i16 2) -> (F-format string=w394:string)  [unwired: 2 in]
    n366 = Number To Fractional String(number=w383, precision (6)=i16 2) -> (F-format string=w393:string)  [unwired: 2 in]
    n367 = Number To Fractional String(number=w382, precision (6)=i16 2) -> (F-format string=w392:string)  [unwired: 2 in]
    n368 = Number To Fractional String(number=w381, precision (6)=i16 2) -> (F-format string=w391:string)  [unwired: 2 in]
    n369 = Number To Fractional String(number=w380, precision (6)=i16 2) -> (F-format string=w390:string)  [unwired: 2 in]
    n370 = Number To Decimal String(number=w463) -> (decimal integer string=w389:string)  [unwired: 1 in]
    n371 = Number To Decimal String(number=w462) -> (decimal integer string=w388:string)  [unwired: 1 in]
    n372 = Build Array(w440, w439, w438, w437, w436, w434, w432, w431, w429, w428, w427, w426, w425, w424, w423, w340, w422, w421, w419, w417, w416, w415, w414, w413, w412, w411, w410, w409, w408, w407, w406, w405, w404, w403, w401, w400, w399, w398, w397, w396, w395, w394, w393, w392, w391, w390, w389, w388, w387, w187, w80, w78, w77, w74, w73, w132, w128, w59, w58, w112, w104, w71, w88, w69, w175, w174, w49, w48, w39) -> (w379:string[])
    n373 = To Unsigned Byte Integer(number=w463) -> (unsigned 8bit integer=w255:u8)
    n374 = To Unsigned Byte Integer(number=w462) -> (unsigned 8bit integer=w254:u8)
    n375 = To Unsigned Byte Integer(number=w435) -> (unsigned 8bit integer=w266:u8)
    n376 = To Unsigned Byte Integer(number=w433) -> (unsigned 8bit integer=w265:u8)
    n377 = To Unsigned Byte Integer(number=w430) -> (unsigned 8bit integer=w264:u8)
    n378 = To Unsigned Byte Integer(number=w420) -> (unsigned 8bit integer=w263:u8)
    n379 = To Unsigned Word Integer(number=w530) -> (unsigned 16bit integer=w257:u16)
    n380 = Bundle By Name(cluster=T1 {"Cycle End Time"=0, "Cycles Run"=0, "Cycle Start Time"=0, "Cycle Knob"="", "Load Type"="", "OOB-Redistrib"=0, "OOB-Fallbacks"=0, "OOB-Retry"=0, "Temp at Start"="", "Load Size At Start"="", "Deep Fill At Start"="", "Soil Level At Start"="", "Spin At Start"="", "Extra rinse At Start"=FALSE, "Deep rinse At Start"=FALSE, "Stain At Start"="", "Soak At Start"="", "Warm Rinse At Start"=FALSE, "Temp at End"="", "Load Size At End"="", "Deep Fill At End"="", "Soil Level At End"="", "Spin At End"="", "Extra rinse At End"=FALSE, "Deep rinse At End"=FALSE, "Stain At End"="", "Soak At End"="", "Warm Rinse At End"=FALSE, "Pauses Count"=0, "Fault Occured"=FALSE, "Delay Flag"=FALSE, "Mycycle Flag"=FALSE, "Blackout"=FALSE, "Cycle completed"=FALSE, "Detected Load Size"=0.0, "Initial Gallons"=0.0, "Last C Inlet "=0.0, "Max Voltage"=0.0, "Target Max Spin"=0, "Max Spin Speed"=0, "Initial Therm"=0.0, "Max Current"=0.0, "Previous Gallons"=0.0, "Initial Water Level"=0.0, "Max Water Level"=0.0, "Abatements "=0, "Lid Open Events"=0, "Cycle Selected"="", "Last H Inlet "=0.0, "WOD-Detg Val Time"=0, "WOD-Total Gallons"=0, "Max Gallons"=0, "Wet Load Gallons"=0, "Gallons at EoC"=0, "Pressure at EoC"=0, "Stk Mnt Water Add"=0, "Started By remote"=FALSE, "Stopped By Remote"=FALSE, "System Reset Count"=0, "Smrt Disp at start"="", "Smrt Disp at EOC"="", "Max Jerk 1st SS"=0, "Max Jerk Final SS"=0, "Max Accelerometer"=0, "Bskt Speed Max Accel"=0, "Max Target Gallons"=0, "Jerk Delta Reject "=0, "Jerk Delta OOB  "=0, "Adaptive Fill Count"=0} ("Cycle History Diagnostics"), "Cycle End Time"=w653, "Cycles Run"=w647, "Cycle Start Time"=w641, "Cycle Knob"=w437, "Load Type"=w436, "OOB-Redistrib"=w266, "OOB-Fallbacks"=w265, "OOB-Retry"=w264, "Temp at Start"=w429, "Load Size At Start"=w428, "Deep Fill At Start"=w427, "Soil Level At Start"=w426, "Spin At Start"=w425, "Extra rinse At Start"=w626, "Deep rinse At Start"=w625, "Stain At Start"=w340, "Soak At Start"=w422, "Warm Rinse At Start"=w621, "Pauses Count"=w263, "Fault Occured"=w589, "Delay Flag"=w271, "Mycycle Flag"=w418, "Blackout"=w588, "Cycle completed"=w587, "Temp at End"=w412, "Load Size At End"=w411, "Deep Fill At End"=w410, "Soil Level At End"=w409, "Spin At End"=w408, "Extra rinse At End"=w604, "Deep rinse At End"=w603, "Stain At End"=w405, "Soak At End"=w404, "Warm Rinse At End"=w602, "Detected Load Size"=w402, "Initial Gallons"=w378, "Last C Inlet"=w386, "Last H Inlet"=w385, "Max Voltage"=w384, "Target Max Spin"=w256, "Max Spin Speed"=w257, "Initial Therm"=w115, "Max Current"=w383, "Previous Gallons"=w382, "Initial Water Level"=w381, "Max Water Level"=w380, "Abatements"=w255, "Lid Open Events"=w254, "Cycle Selected"=w387, "WOD-Detg Val Time"=w185, "WOD-Total Gallons"=w166, "Max Gallons"=w158, "Wet Load Gallons"=w145, "Gallons at EoC"=w135, "Pressure at EoC"=w136, "Stk Mnt Water Add"=w131, "Started By remote"=w173, "Stopped By Remote"=w165, "System Reset Count"=w127, "Smrt Disp at start"=w59, "Smrt Disp at EOC"=w58, "Max Jerk 1st SS"=w111, "Max Jerk Final SS"=w103, "Max Accelerometer"=w90, "Bskt Speed Max Accel"=w87, "Max Target Gallons"=w82, "Jerk Delta Reject"=w47, "Jerk Delta OOB"=w46, "Adaptive Fill Count"=w40) -> (w441:T1)
  }
  "Cycle  Diag Array Out" <- w3
  n381 = Bundle By Name(cluster=T2 {"Current Index"=0, "Count"=0, "Overwrite Count"=0} ("Cycle Buffer Status"), "Current Index"=w28, "Count"=w10, "Overwrite Count"=w29) -> (→"Cycle Buffer Status":T2)
  n382 = Transpose 2D Array(2D array=w2) -> (transposed array=→"Diag Cycle String Out":string[][])
